vi "MakeDataFileForMultiplot.vi"(4 "Y Axis Name":string, 5 "Plot Array":cluster{"Angle":dbl[], "Radius":dbl[]}[](array[cluster]), 6 "X Axis Name":string, 7 "Path":path, 9 "Transpose":bool, 10 "Plot Summary":string[][](array[string]), 11 "Legend":string[](array[string])) -> ()   [LabVIEW 2013]
uses:
  Results_plotter_Global.vi
panel:
  out "datLoops":i32
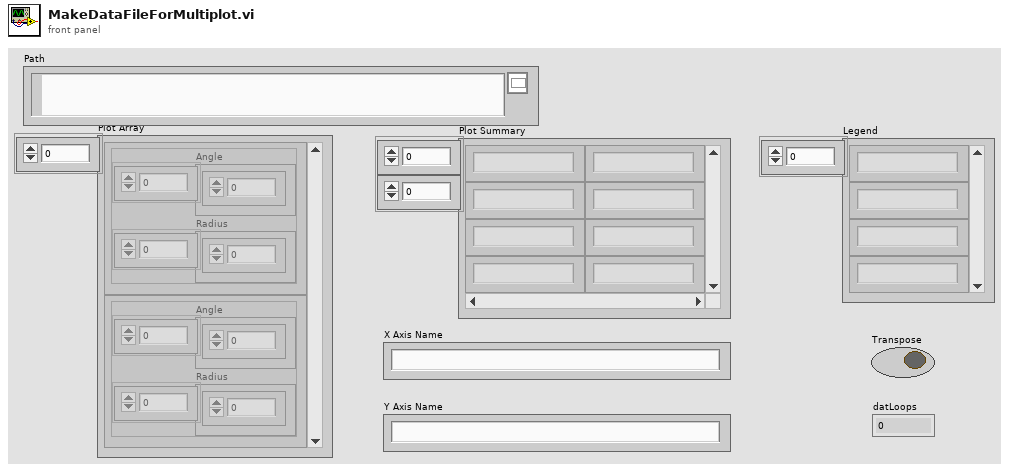
[diagram p1: front panel]
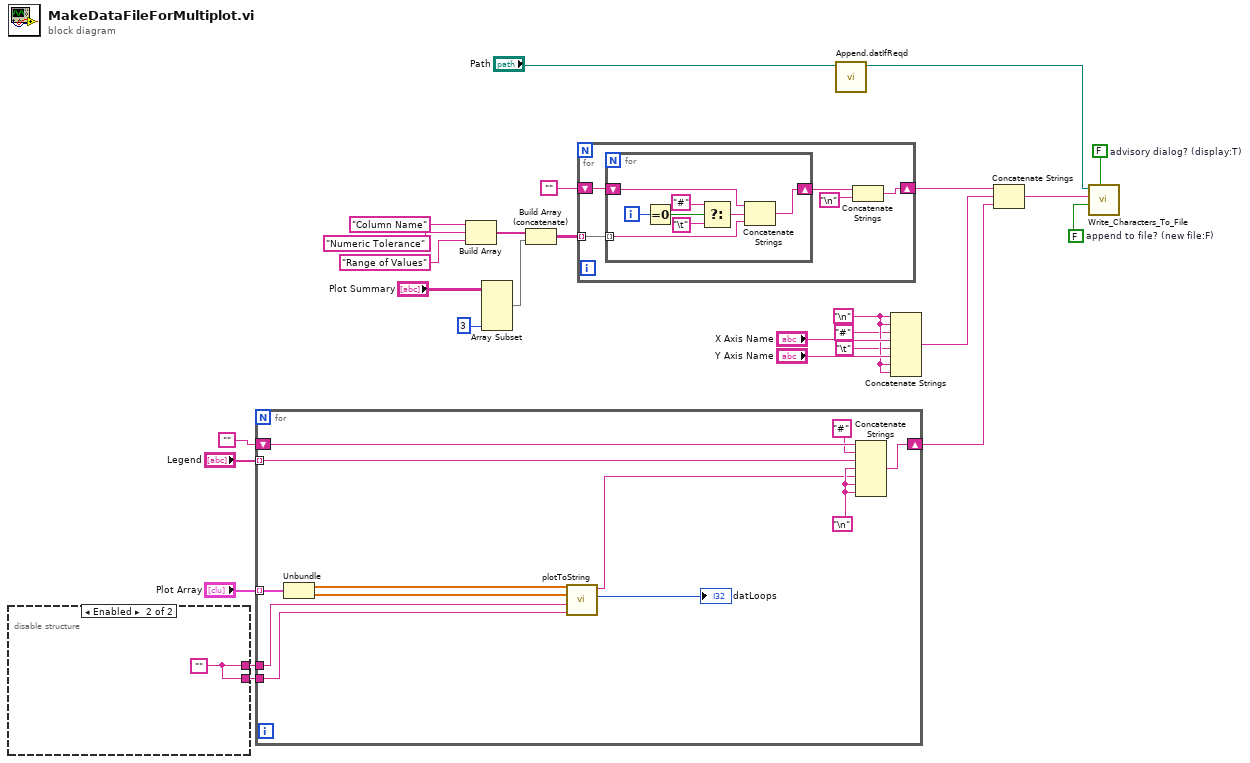
[diagram p0: block diagram]
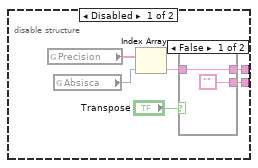
[diagram p2: hidden frame]
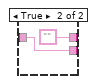
[diagram p3: hidden frame]
diagram:
  w7 = FALSE  # advisory dialog? (display:T)
  w6 = FALSE  # append to file? (new file:F)
  w16 = "\n"
  n1 = disable-structure shown="Enabled" {
    disable-tunnel: [w29 w38] -> w10
    disable-tunnel: [w28 w38] -> w9
    frame Disabled {
      n2 = global read "Results_plotter_Global.vi" "Precision"() -> (w30:string[])
      n3 = global read "Results_plotter_Global.vi" "Absisca"() -> (w31:i32)
      n4 = Index Array(array=w30, index=w31) -> (element=w32:string)
      n5 = case shown="False" "Transpose" {
        tunnel: ["" w37] -> w28
        tunnel: w32 -> [w34 w37]
        tunnel: [w34 ""] -> w29
        frame False {
        }
        frame True {
        }
      }
    }
    frame Enabled {
      w38 = ""
    }
  }
  n6 = for {
    tunnel: "Plot Array" -> [w50] mode=indexing
    shift-right: [w49] -> w2
    shift-left: "" -> [w44]
    tunnel: "Legend" -> [w42] mode=indexing
    tunnel: w10 -> [w41]
    tunnel: w9 -> [w39]
    w48 = "\n"
    n7 = Unbundle(w50) -> ("Angle"=w45:dbl[], "Radius"=w46:dbl[])
    n8 = call "plotToString.vi"("Precision2"=w39, "Precision1"=w41, "Column2"=w46, "Column1"=w45) -> ("nLoops"=→"datLoops":i32, "plotString"=w47:string)  [unwired: 6 in]
    n9 = Concatenate Strings(w44, "#", w42, w48, w47, w48, w48) -> (w49:string)
  }
  n10 = Build Array("Column Name", "Numeric Tolerance", "Range of Values") -> (w19:string[])
  n11 = Array Subset(array="Plot Summary", length (col)=3 ("length")) -> (w24:string[][])  [unwired: 3 in]
  n12 = Build Array (concatenate)(w19, w24) -> (w26:string[][])
  n13 = for {
    shift-right: [w54] -> w4
    shift-left: "" -> [w51]
    tunnel: w26 -> [w55] mode=indexing
    n14 = for {
      shift-right: [w56] -> w53
      shift-left: w51 -> [w63]
      tunnel: w55 -> [w57] mode=indexing
      i -> [w62]
      n15 = Equal To 0?(x=w62) -> (x = 0?=w61:bool)
      n16 = Select(t="#", s=w61, f="\t") -> (s? t:f=w58:string)
      n17 = Concatenate Strings(w63, w58, w57) -> (w56:string)
    }
    n18 = Concatenate Strings(w53, "\n") -> (w54:string)
  }
  n19 = call "Append.datIfReqd.vi"("Path"="Path") -> ("appended path"=w8:path)  [unwired: 10 in]
  n20 = Concatenate Strings(w16, w16, "#" ("string"), "X Axis Name", "\t", "Y Axis Name", w16, w16) -> (w3:string)
  n21 = Concatenate Strings(w4, w3, w2) -> (w5:string)
  n22 = call "Write_Characters_To_File.vi"("file path (dialog if empty)"=w8, "advisory dialog? (display:T)"=w7, "character string"=w5, "append to file? (new file:F)"=w6) -> ()  [unwired: 1 in, 4 out]
